vi "SUB_SearchFile_inFolder.vi"(2 "Search Filename in Folder":string) -> (0 "File Existing True/Flase":bool)   [LabVIEW 2011]
panel:
  out "error out":errorcluster
  out "spreadsheet string":string
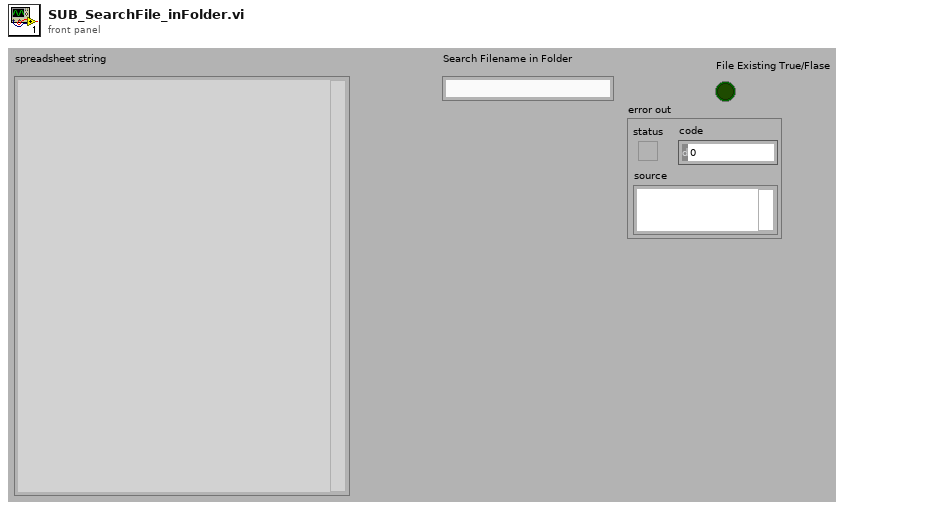
[diagram p1: front panel]
types:
  T1 = enum32{"invalid app kind", "Development System", "Run Time System", "Student Edition", "Embedded LabVIEW", "Evaluation", "Custom"}
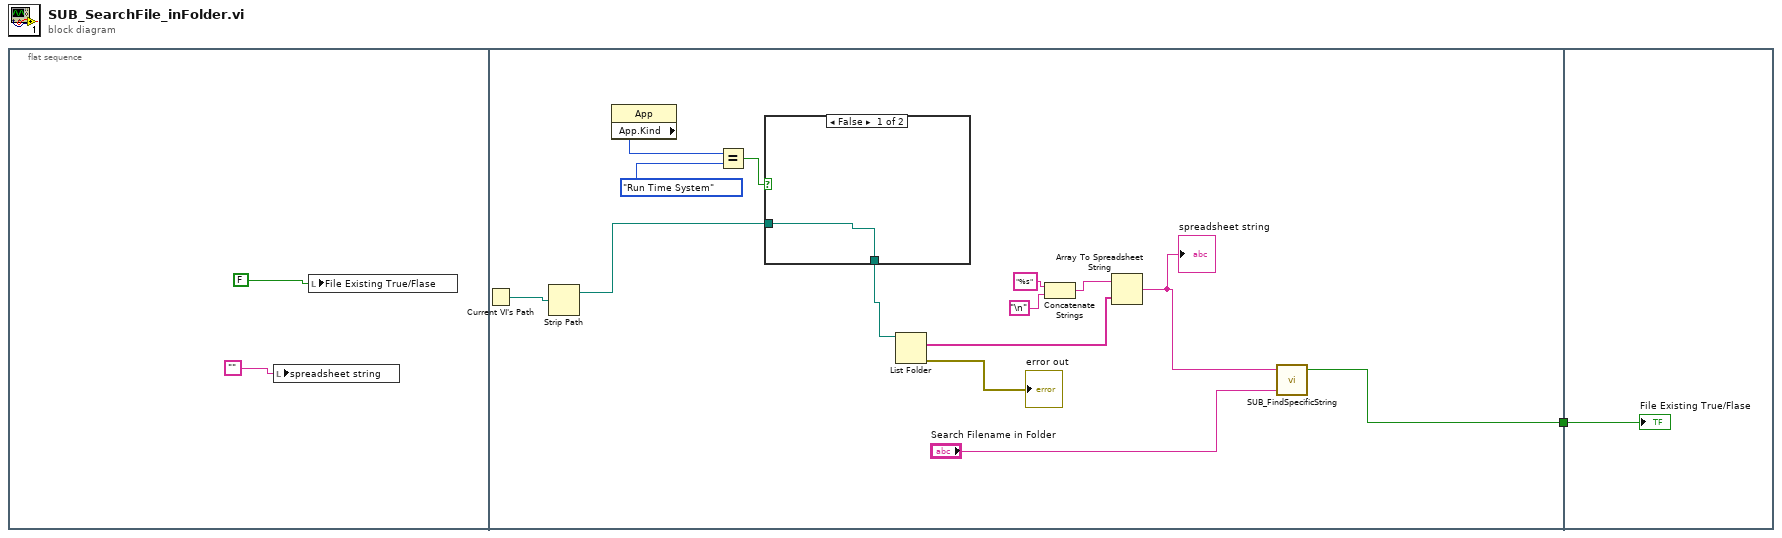
[diagram p0: block diagram]
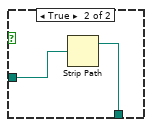
[diagram p2: hidden frame]
diagram:
  n1 = flat-sequence {
    tunnel: [w4] -> w1
    tunnel: w1 -> [w21]
    frame #0 {
      n2 = local write "spreadsheet string"("") -> ()
      n3 = local write "File Existing True/Flase"(FALSE) -> ()
    }
    frame #1 {
      n4 = Current VI's Path() -> (path=w17:path)
      n5 = Strip Path(path=w17) -> (stripped path=w13:path)  [unwired: 1 out]
      n6 = property class="App"() -> ("App.Kind"=w14:T1)  [unwired: 2 in, 2 out]
      n7 = Equal?(x=w14, y=T1."Run Time System" ("Application:Kind")) -> (x = y?=w16:bool)
      n8 = case shown="False" w16 {
        tunnel: [w18 w20] -> w12
        tunnel: w13 -> [w18 w19]
        frame False {
        }
        frame True {
          n9 = Strip Path(path=w19) -> (stripped path=w20:path)  [unwired: 1 out]
        }
      }
      n10 = List Folder(path=w12) -> (filenames=w11:string[], error out=→"error out":errorcluster)  [unwired: 3 in, 2 out]
      n11 = Concatenate Strings("%s" ("format string"), "\n") -> (w8:string)
      n12 = Array To Spreadsheet String(array=w11, 3:w8) -> (spreadsheet string=w6:string)  [unwired: 1 in]
      "spreadsheet string" <- w6
      n13 = call "SUB_FindSpecificString.vi"("Find this String"="Search Filename in Folder", "String data"=w6) -> ("Found"=w4:bool)  [unwired: 2 in, 1 out]
    }
    frame #2 {
      "File Existing True/Flase" <- w21
    }
  }
